vi "pic and ftp.vi"(11 "To: 2":string="pankaj7897@outlook.com") -> (3 "Image Out":T1(plugin-control))   [LabVIEW 2013]
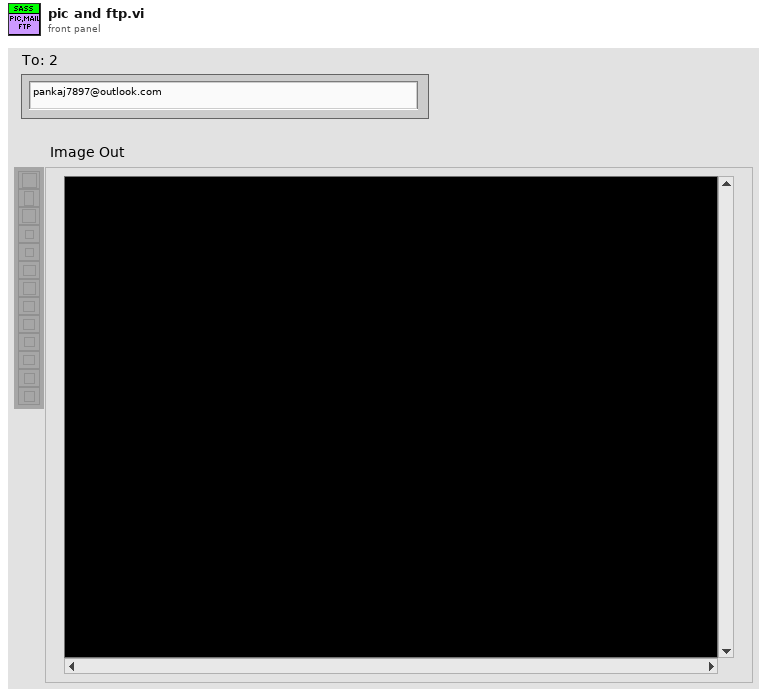
[diagram p1: front panel]
types:
  T1 = typedef "IMAQ Image.ctl" = refnum<image>
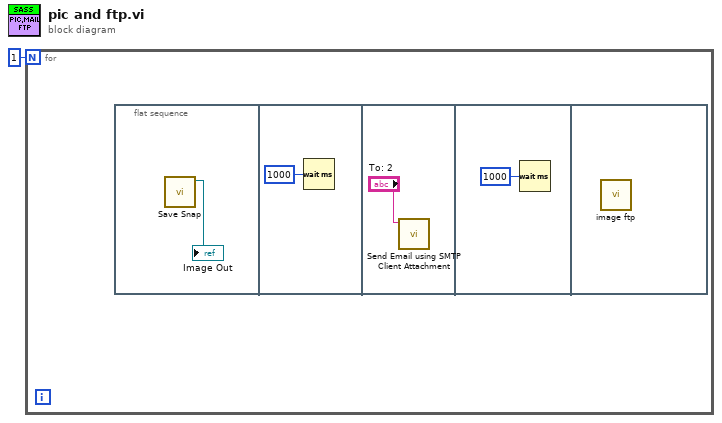
[diagram p0: block diagram]
diagram:
  n1 = for {
    N: 1 -> [_]
    n2 = flat-sequence {
      frame #0 {
        n3 = call "Save Snap.vi"() -> ("Image Out"=→"Image Out":T1)  [unwired: 11 in]
      }
      frame #1 {
        n4 = Wait (ms)(milliseconds to wait=u32 1000) -> ()  [unwired: 1 out]
      }
      frame #2 {
        n5 = call "Send Email using SMTP Client Attachment.vi"("To: 2"="To: 2") -> ()  [unwired: 11 in]
      }
      frame #3 {
        n6 = Wait (ms)(milliseconds to wait=u32 1000) -> ()  [unwired: 1 out]
      }
      frame #4 {
        n7 = call "image ftp.vi"() -> ()  [unwired: 12 in]
      }
    }
  }
